vi "_API_BINANCE_GET_CashOnAccount.vi"(0 "BinanceAPI in":refnum<class "BinanceAPI_.lvclass">, 5 "CashOnAccount":cluster{"Symbol (BTC)":string}, 11 "error in (no error)":errorcluster) -> (4 "BinanceAPI out":refnum<class "BinanceAPI_.lvclass">, 6 "CashOnAccount_Data":cluster{"Free":ext, "Locked":ext}={"Free"=nan, "Locked"=nan}, 14 "Body":string, 15 "error out":errorcluster)   [LabVIEW 2022 SP3, in "BinanceAPI_.lvclass"]
doc: "https://binance-docs.github.io/apidocs/spot/en/#account-information-user_data"
uses:
  BinanceAPI_.lvclass
  BinanceAPI_.lvclass/BinanceAPI_.ctl
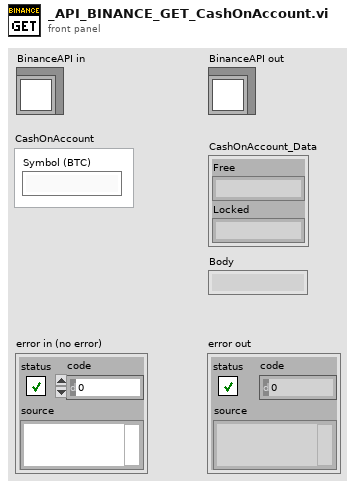
[diagram p1: front panel]
types:
  T1 = enum16{"SPOT", "USDT_FUTURES", "COIN_FUTURES", "VANILLA"}
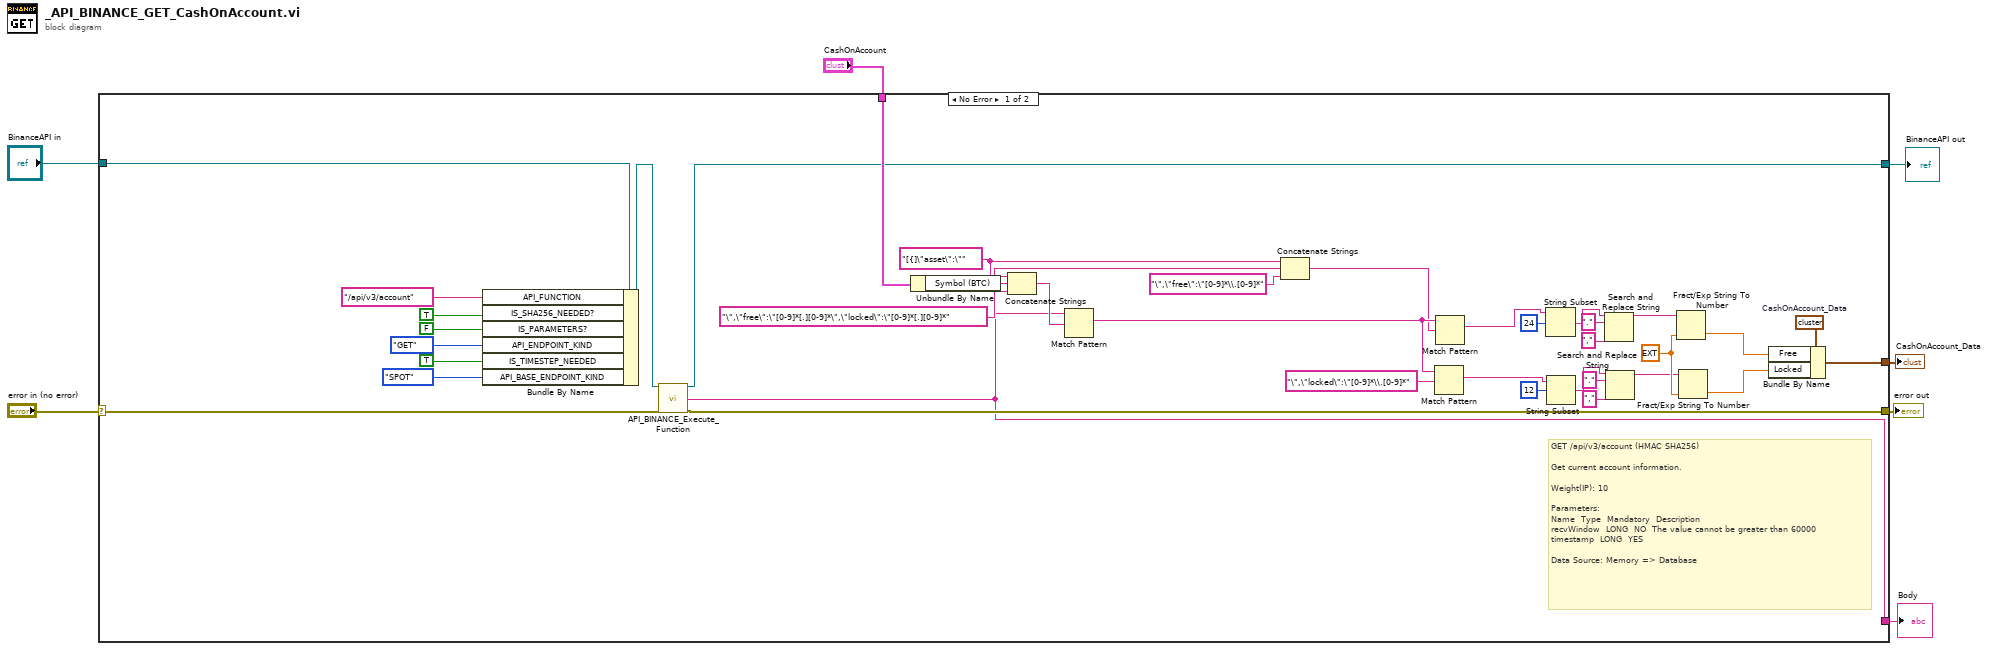
[diagram p0: block diagram]
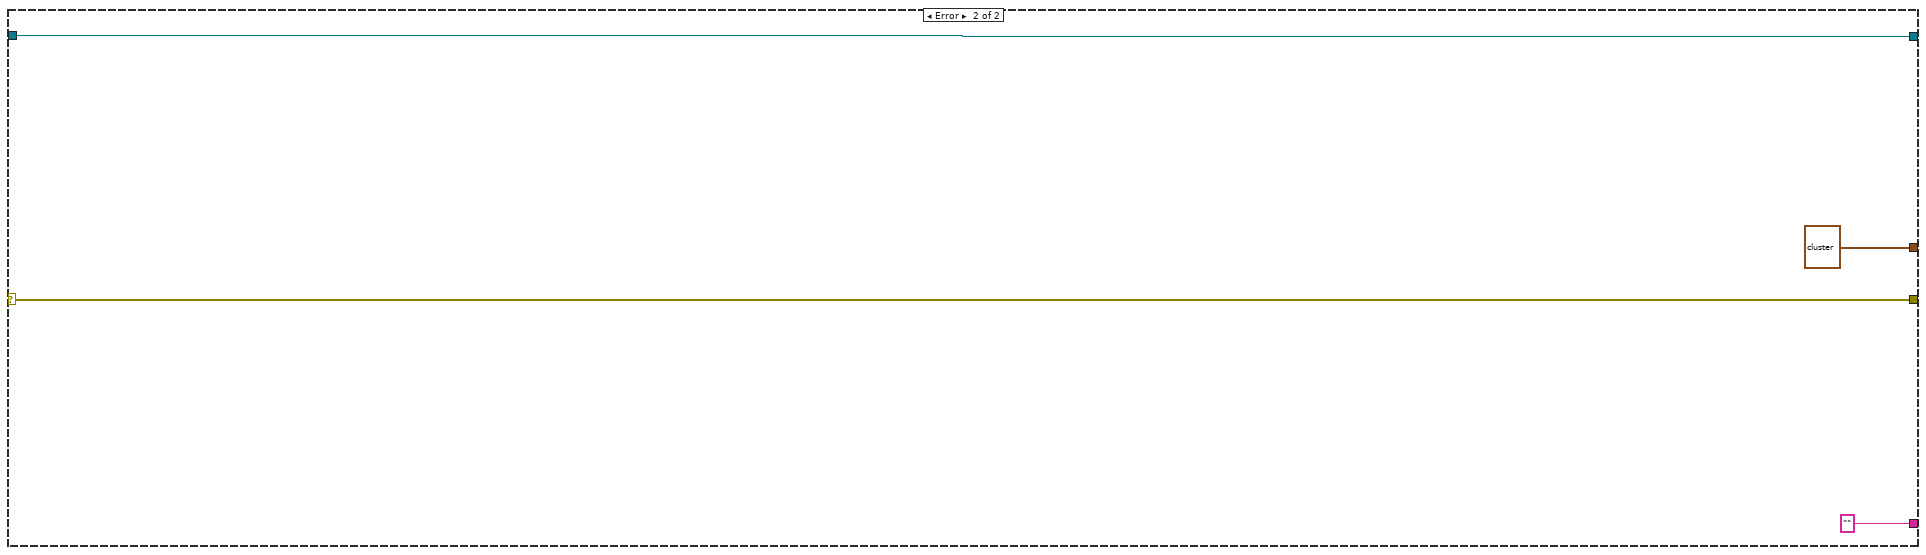
[diagram p2: hidden frame]
diagram:
  n1 = case shown="No Error" "error in (no error)" {
    selector: "error in (no error)" -> [w12 w49]
    tunnel: [w13 w49] -> w6
    tunnel: [w14 w48] -> w2
    tunnel: "BinanceAPI in" -> [w11 w48]
    tunnel: "CashOnAccount" -> [w39 _]
    tunnel: [w17 cluster{"Free":ext, "Locked":ext} {"Free"=nan, "Locked"=nan} ("CashOnAccount_Data")] -> w4
    tunnel: [w8 "" ("Body")] -> w3
    frame No Error {
      w20 = cluster{"Free":ext, "Locked":ext} {"Free"=0.0, "Locked"=0.0}  # CashOnAccount_Data
      w28 = ext 0.0
      w36 = "[{]\"asset\":\""
      # "GET /api/v3/account (HMAC SHA256)\n\nGet current account information.\n\nWeight(IP): 10\n\nParameters:\nName \tType \tMandatory \tDescription\nrecvWindow \tLONG \tNO \tThe value cannot be greater than 60000\ntimestamp \tLONG \tYES \t\n\nData Source: Memory => Database"
      n2 = Bundle By Name(cluster=w11, "API_FUNCTION"="/api/v3/account", "IS_SHA256_NEEDED?"=TRUE, "IS_PARAMETERS?"=FALSE, "API_ENDPOINT_KIND"=enum16{"POST", "DELETE", "GET", "PUT"}."GET", "IS_TIMESTEP_NEEDED"=TRUE, "API_BASE_ENDPOINT_KIND"=T1."SPOT") -> (w15:refnum<class "BinanceAPI_.lvclass">)
      n3 = call "API_BINANCE_Execute_Function.vi"("BinanceAPI in"=w15, "error in (no error)"=w12) -> ("BinanceAPI out"=w14:refnum<class "BinanceAPI_.lvclass">, "Body"=w8:string, "error out"=w13:errorcluster)  [unwired: 9 in, 2 out]
      n4 = Unbundle By Name(w39) -> ("Symbol (BTC)"=w35:string)
      n5 = Concatenate Strings(w36, w35, "\",\"free\":\"[0-9]*[.][0-9]*\",\"locked\":\"[0-9]*[.][0-9]*") -> (w40:string)
      n6 = Match Pattern(string=w8, regular expression=w40) -> (match substring=w38:string)  [unwired: 1 in, 3 out]
      n7 = Concatenate Strings(w36, w35, "\",\"free\":\"[0-9]*\\.[0-9]*") -> (w33:string)
      n8 = Match Pattern(string=w38, regular expression="\",\"locked\":\"[0-9]*\\.[0-9]*") -> (match substring=w32:string)  [unwired: 1 in, 3 out]
      n9 = Match Pattern(string=w38, regular expression=w33) -> (match substring=w29:string)  [unwired: 1 in, 3 out]
      n10 = String Subset(string=w29, offset (0)=24) -> (substring=w27:string)  [unwired: 1 in]
      n11 = String Subset(string=w32, offset (0)=12) -> (substring=w21:string)  [unwired: 1 in]
      n12 = Search and Replace String(input string=w27, search string=".", replace string="," ("replace string (\"\")")) -> (result string=w24:string)  [unwired: 5 in, 3 out]
      n13 = Search and Replace String(input string=w21, search string=".", replace string="," ("replace string (\"\")")) -> (result string=w16:string)  [unwired: 5 in, 3 out]
      n14 = Fract/Exp String To Number(string=w24, default (0 dbl)=w28) -> (number=w19:ext)  [unwired: 2 in, 1 out]
      n15 = Fract/Exp String To Number(string=w16, default (0 dbl)=w28) -> (number=w18:ext)  [unwired: 2 in, 1 out]
      n16 = Bundle By Name(cluster=w20, "Free"=w19, "Locked"=w18) -> (w17:cluster{"Free":ext, "Locked":ext})
    }
    frame Error {
    }
  }
  "error out" <- w6
  "CashOnAccount_Data" <- w4
  "Body" <- w3
  "BinanceAPI out" <- w2
